vi "Configure Auto Zero.vi"(8 "error in (no error)":errorcluster, 9 "Zero Type (0: External)":i32(ring) items=["External", "Internal"], 10 "Auto Zero (T: Enable)":bool=TRUE, 11 "VISA resource name":refnum<visa-resource-name>) -> (0 "error out":errorcluster, 3 "VISA resource name out":refnum<visa-resource-name>)   [LabVIEW 2014, in "Agilent U2000 Series.lvlib"]
doc: "Enables or disables auto zero."
uses:
  Agilent U2000 Series.lvlib
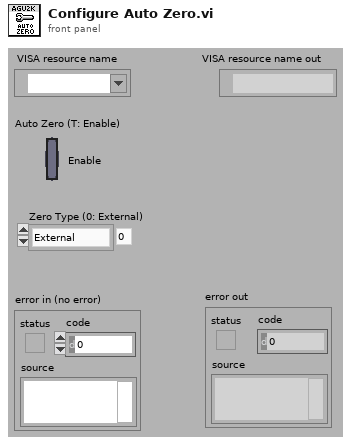
[diagram p1: front panel]
types:
  T1 = typedef "Agilent U2000 Series.lvlib/Extended User Data.ctl" = cluster{"U2000 Series Mode":u16, "Trigger Source Int/Ext":bool}
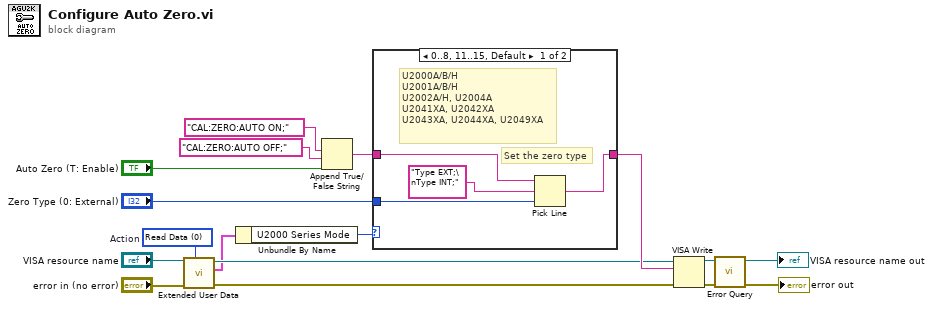
[diagram p0: block diagram]
diagram:
  w2 = 0 items=["Read Data", "Write Data", "Clear Data", "Clear ALL Data"]  # Action
  n1 = call "Extended User Data.vi"("Action (1: Write Data)"=w2, "error in (no error)"="error in (no error)", "VISA resource name"="VISA resource name") -> ("error out"=w5:errorcluster, "User Data Out"=w4:T1, "VISA resource name out"=w6:refnum<visa-resource-name>)  [unwired: 1 in, 5 out]
  n2 = Unbundle By Name(w4) -> ("U2000 Series Mode"=w3:u16)
  n3 = Append True/False String(1:"Auto Zero (T: Enable)", 2:"CAL:ZERO:AUTO OFF;", 3:"CAL:ZERO:AUTO ON;") -> (0:w11:string)  [unwired: 1 out]
  n4 = case shown="0..8, 11..15, Default" w3 {
    tunnel: w11 -> [w21 w22]
    tunnel: [w18 w22] -> w10
    tunnel: "Zero Type (0: External)" -> [w19 _]
    frame 0..8, 11..15, Default {
      # "U2000A/B/H\nU2001A/B/H\nU2002A/H, U2004A\nU2041XA, U2042XA\nU2043XA, U2044XA, U2049XA"
      # "Set the zero type"
      n5 = Pick Line(string ("")=w21, multi-line string="Type EXT;\nType INT;", line index=w19) -> (output string=w18:string)
    }
    frame 9, 10 {
      # "U2021XA\nU2022XA"
    }
  }
  n6 = VISA Write(VISA resource name=w6, write buffer=w10, error in (no error)=w5) -> (VISA resource name out=w14:refnum<visa-resource-name>, error out=w13:errorcluster)  [unwired: 1 out]
  n7 = call "Error Query.vi"("error in (no error)"=w13, "VISA resource name"=w14) -> ("error out"=→"error out":errorcluster, "VISA resource name out"=→"VISA resource name out":refnum<visa-resource-name>)  [unwired: 8 out]
